vi "Load Yaml.vi"(8 "error in (no error)":errorcluster, 11 "Yaml Model in":refnum<class "Yaml Model.lvclass">) -> (0 "error out":errorcluster, 3 "Yaml Model out":refnum<class "Yaml Model.lvclass">)   [LabVIEW 2020, in "Yaml Model.lvlib" / "Yaml Model.lvclass"]
uses:
  Yaml Model.lvclass
  Yaml Model.lvclass/Yaml Model.ctl
panel:
  # "NOTICE -- YOU MUST LEAVE THIS NOTICE IN PLACE.\n\nCopyright (c) 2017, LIANG LIU Shawn.Liu.cn@gmail.com\nAll rights reserved.\n\nRedistribution and use in source and binary forms, with or without modification, are permitted provided that the following conditions are met:\n-Redistributions of source code must retain the above copyright notice, this list of conditions and the following disclaimer.\n-Redistributions in binary form must reproduce the above copyright notice, this list of conditions and the following disclaimer in the documentation and/or other materials provided with the distribution.\n-Neither the name of the eLp nor the names of its contributors may be used to endorse or promote products derived from this software without specific prior written permission.\n\nTHIS SOFTWARE IS PROVIDED BY THE COPYRIGHT HOLDERS AND CONTRIBUTORS \"AS IS\" AND ANY EXPRESS OR IMPLIED WARRANTIES, INCLUDING, BUT NOT LIMITED TO, THE IMPLIED WARRANTIES OF MERCHANTABILITY AND FITNESS FOR A PARTICULAR PURPOSE ARE DISCLAIMED. IN NO EVENT SHALL THE COPYRIGHT HOLDER OR CONTRIBUTORS BE LIABLE FOR ANY DIRECT, INDIRECT, INCIDENTAL, SPECIAL, EXEMPLARY, OR CONSEQUENTIAL DAMAGES (INCLUDING, BUT NOT LIMITED TO, PROCUREMENT OF SUBSTITUTE GOODS OR SERVICES; LOSS OF USE, DATA, OR PROFITS; OR BUSINESS INTERRUPTION) HOWEVER CAUSED AND ON ANY THEORY OF LIABILITY, WHETHER IN CONTRACT, STRICT LIABILITY, OR TORT (INCLUDING NEGLIGENCE OR OTHERWISE) ARISING IN ANY WAY OUT OF THE USE OF THIS SOFTWARE, EVEN IF ADVISED OF THE POSSIBILITY OF SUCH DAMAGE."
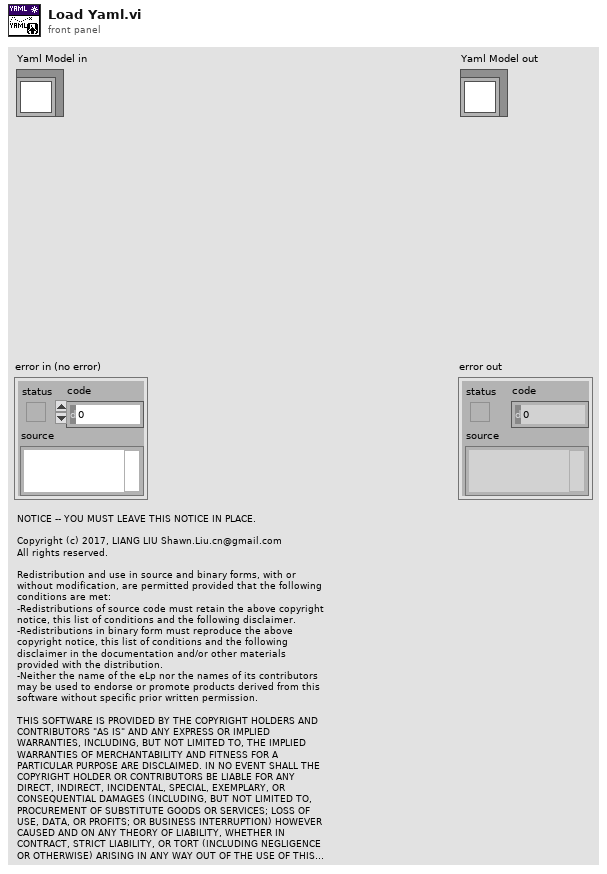
[diagram p1: front panel]
types:
  T1 = enum8{"Enabled", "Disabled", "Disabled and Grayed Out"}
  T2 = cluster{"Image":string, "Resolution":dbl, "Origin":cluster{"X":dbl, "Y":dbl, "R":dbl}, "Occupied Thresh":dbl, "Free Thresh":dbl, "Negate":bool}
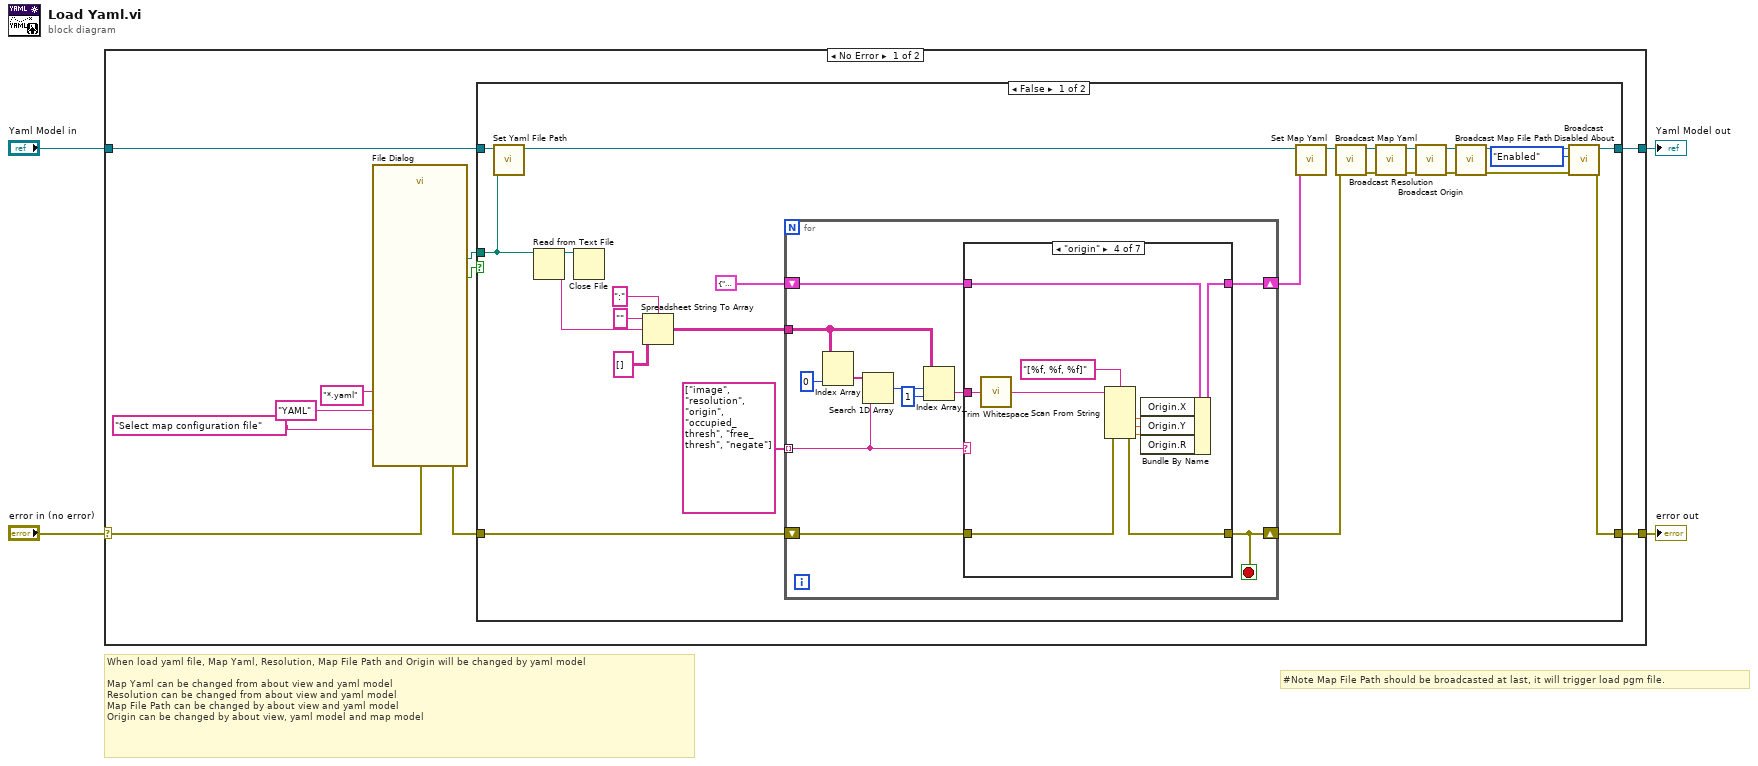
[diagram p0: block diagram]
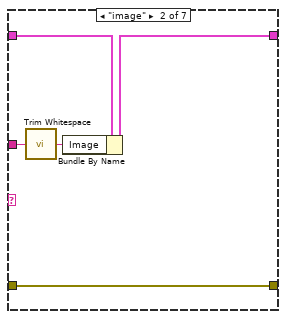
[diagram p3: hidden frame]
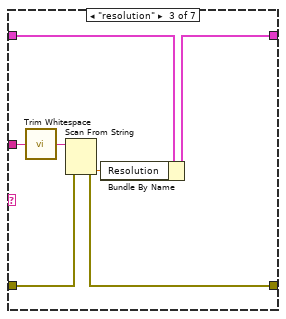
[diagram p4: hidden frame]
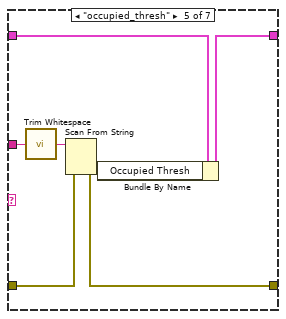
[diagram p5: hidden frame]
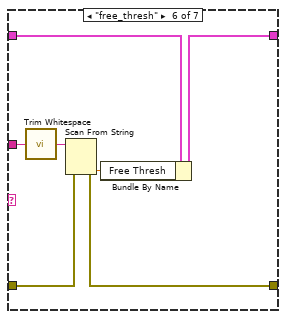
[diagram p6: hidden frame]
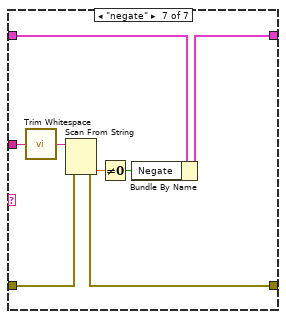
[diagram p7: hidden frame]
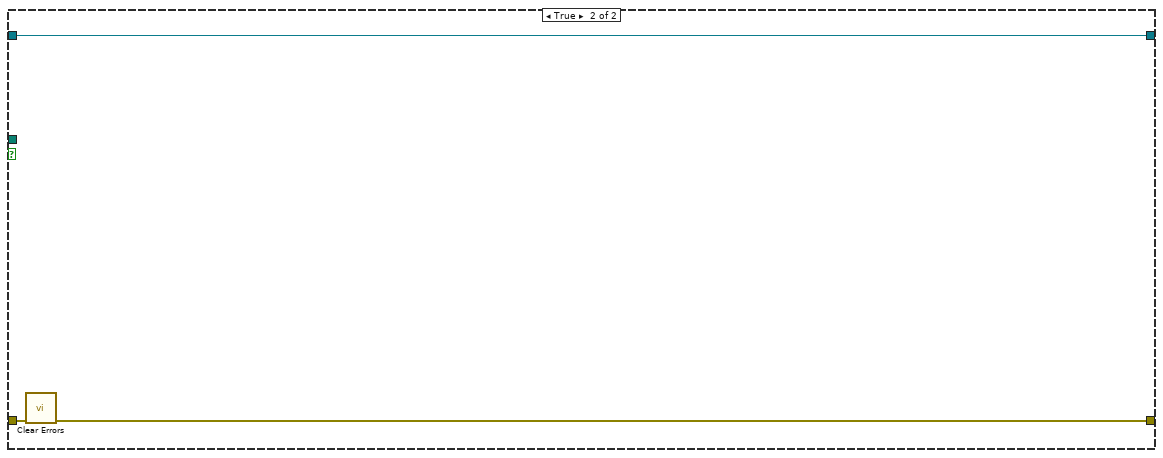
[diagram p8: hidden frame]
diagram:
  # "#Note Map File Path should be broadcasted at last, it will trigger load pgm file."
  # "When load yaml file, Map Yaml, Resolution, Map File Path and Origin will be changed by yaml model\n\nMap Yaml can be changed from about view and yaml model\nResolution can be changed from about view and yaml model\nMap File Path can be changed by about view and yaml model\nOrigin can be changed by about view, yaml model and map model"
  n1 = case shown="No Error" "error in (no error)" {
    selector: "error in (no error)" -> [w12 w102]
    tunnel: "Yaml Model in" -> [w14 w101]
    tunnel: [w13 w101] -> w3
    tunnel: [w11 w102] -> w1
    frame No Error {
      n2 = call "File Dialog"("prompt"="Select map configuration file", "error in"=w12, "pattern (all files)"="*.yaml", "pattern label"="YAML") -> ("selected path"=w6:path, "cancelled"=w7:bool, "error out"=w5:errorcluster)  [unwired: 8 in, 1 out]
      n3 = case shown="False" w7 {
        tunnel: w14 -> [w40 w100]
        tunnel: [w25 w100] -> w13
        tunnel: w6 -> [w37 _]
        tunnel: w5 -> [w28 w99]
        tunnel: [w15 w98] -> w11
        frame False {
          n4 = call "Set Yaml File Path.vi"("Yaml File Path"=w37, "Yaml Model in"=w40) -> ("Yaml Model out"=w38:refnum<class "Yaml Model.lvclass">)  [unwired: 9 in]
          n5 = Read from Text File(file (use dialog)=w37) -> (refnum out=w39:refnum<file>, text=w31:string)  [unwired: 3 in, 2 out]
          n6 = Close File(refnum=w39) -> ()  [unwired: 1 in, 2 out]
          n7 = Spreadsheet String To Array(delimiter (Tab)=":", format string="", spreadsheet string=w31, array type (2D Dbl)=string[][] []) -> (array=w33:string[][])
          n8 = for {
            tunnel: w33 -> [w48]
            tunnel: string[] ["image", "resolution", "origin", "occupied_thresh", "free_thresh", "negate"] -> [w43] mode=indexing
            shift-right: [w45] -> w29
            shift-left: T2 {"Image"="", "Resolution"=0.0, "Origin"={"X"=0.0, "Y"=0.0, "R"=0.0}, "Occupied Thresh"=0.0, "Free Thresh"=0.0, "Negate"=FALSE} ("Map Yaml") -> [w46]
            shift-right: [w41] -> w16
            shift-left: w28 -> [w42]
            stop <- w41 stop-if-true
            n9 = Index Array(array=w48, index (col)=0 ("disabled index (col)")) -> (element=w51:string[])  [unwired: 1 in]
            n10 = Search 1D Array(1D array=w51, element=w43) -> (index of element=w50:i32)  [unwired: 1 in]
            n11 = Index Array(array=w48, index (row)=w50, index (col)=1 ("disabled index (col)")) -> (element=w44:string)
            n12 = case shown="\"origin\"" w43 {
              tunnel: w46 -> [w53 w58 w65 w75 w82 w89 w97]
              tunnel: [w53 w57 w64 w74 w81 w88 w96] -> w45
              tunnel: w44 -> [_ w56 w63 w73 w80 w87 w95]
              tunnel: w42 -> [w52 w54 w60 w67 w77 w84 w91]
              tunnel: [w52 w54 w59 w66 w76 w83 w90] -> w41
              frame Default {
              }
              frame "image" {
                n13 = call <vilib>:"Trim Whitespace.vi"("string"=w56) -> ("trimmed string"=w55:string)  [unwired: 1 in]
                n14 = Bundle By Name(cluster=w58, "Image"=w55) -> (w57:T2)
              }
              frame "resolution" {
                n15 = call <vilib>:"Trim Whitespace.vi"("string"=w63) -> ("trimmed string"=w61:string)  [unwired: 1 in]
                n16 = Scan From String(input string=w61, error in=w60) -> (error out=w59:errorcluster, output 1=w62:dbl)  [unwired: 3 in, 2 out]
                n17 = Bundle By Name(cluster=w65, "Resolution"=w62) -> (w64:T2)
              }
              frame "origin" {
                n18 = call <vilib>:"Trim Whitespace.vi"("string"=w73) -> ("trimmed string"=w68:string)  [unwired: 1 in]
                n19 = Scan From String(format string="[%f, %f, %f]", input string=w68, error in=w67) -> (error out=w66:errorcluster, output 1=w71:dbl, output 2=w70:dbl, output 3=w69:dbl)  [unwired: 4 in, 2 out]
                n20 = Bundle By Name(cluster=w75, "Origin.X"=w71, "Origin.Y"=w70, "Origin.R"=w69) -> (w74:T2)
              }
              frame "occupied_thresh" {
                n21 = call <vilib>:"Trim Whitespace.vi"("string"=w80) -> ("trimmed string"=w78:string)  [unwired: 1 in]
                n22 = Scan From String(input string=w78, error in=w77) -> (error out=w76:errorcluster, output 1=w79:dbl)  [unwired: 3 in, 2 out]
                n23 = Bundle By Name(cluster=w82, "Occupied Thresh"=w79) -> (w81:T2)
              }
              frame "free_thresh" {
                n24 = call <vilib>:"Trim Whitespace.vi"("string"=w87) -> ("trimmed string"=w85:string)  [unwired: 1 in]
                n25 = Scan From String(input string=w85, error in=w84) -> (error out=w83:errorcluster, output 1=w86:dbl)  [unwired: 3 in, 2 out]
                n26 = Bundle By Name(cluster=w89, "Free Thresh"=w86) -> (w88:T2)
              }
              frame "negate" {
                n27 = call <vilib>:"Trim Whitespace.vi"("string"=w95) -> ("trimmed string"=w93:string)  [unwired: 1 in]
                n28 = Scan From String(input string=w93, error in=w91) -> (error out=w90:errorcluster, output 1=w94:dbl)  [unwired: 3 in, 2 out]
                n29 = Not Equal To 0?(x=w94) -> (x != 0?=w92:bool)
                n30 = Bundle By Name(cluster=w97, "Negate"=w92) -> (w96:T2)
              }
            }
          }
          n31 = call "Set Map Yaml.vi"("Map Yaml"=w29, "Yaml Model in"=w38) -> ("Yaml Model out"=w27:refnum<class "Yaml Model.lvclass">)  [unwired: 9 in]
          n32 = call "Broadcast Map Yaml.vi"("error in (no error)"=w16, "Yaml Model in"=w27) -> ("error out"=w23:errorcluster, "Yaml Model out"=w26:refnum<class "Yaml Model.lvclass">)  [unwired: 8 in]
          n33 = call "Broadcast Resolution.vi"("error in (no error)"=w23, "Yaml Model in"=w26) -> ("error out"=w21:errorcluster, "Yaml Model out"=w22:refnum<class "Yaml Model.lvclass">)  [unwired: 8 in]
          n34 = call "Broadcast Origin.vi"("error in (no error)"=w21, "Yaml Model in"=w22) -> ("error out"=w19:errorcluster, "Yaml Model out"=w20:refnum<class "Yaml Model.lvclass">)  [unwired: 8 in]
          n35 = call "Broadcast Map File Path.vi"("error in (no error)"=w19, "Yaml Model in"=w20) -> ("error out"=w17:errorcluster, "Yaml Model out"=w18:refnum<class "Yaml Model.lvclass">)  [unwired: 8 in]
          n36 = call "Broadcast Disabled About.vi"("error in (no error)"=w17, "Disabled About"=T1."Enabled", "Yaml Model in"=w18) -> ("error out"=w15:errorcluster, "Yaml Model out"=w25:refnum<class "Yaml Model.lvclass">)  [unwired: 7 in]
        }
        frame True {
          n37 = call <vilib>:"Clear Errors.vi"("error in (no error)"=w99) -> ("error out"=w98:errorcluster)  [unwired: 5 in, 1 out]
        }
      }
    }
    frame Error {
    }
  }
  "error out" <- w1
  "Yaml Model out" <- w3
